vi "GetType.vi"(8 "error in (no error)":errorcluster, 11 "Initiate Generation Msg in":refnum<class "Initiate Generation Msg.lvclass">) -> (0 "error out":errorcluster, 2 "Data Sample":variant, 3 "Initiate Generation Msg out":refnum<class "Initiate Generation Msg.lvclass">)   [LabVIEW 2014, in "CS++Fgen.lvlib" / "Initiate Generation Msg.lvclass"]
doc: "This VI delivers a sample of the data type format the message expects."
uses:
  Initiate Generation Msg.lvclass
  Initiate Generation Msg.lvclass/Initiate Generation Msg.ctl
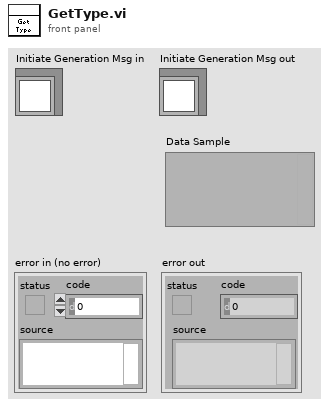
[diagram p1: front panel]
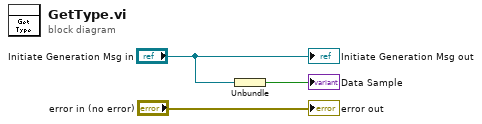
[diagram p0: block diagram]
diagram:
  n1 = Unbundle("Initiate Generation Msg in") -> (→"Data Sample":bool)
  "error out" <- "error in (no error)"
  "Initiate Generation Msg out" <- "Initiate Generation Msg in"
